vi "Pixel Manipulation.vi"() -> (3 "ImgOut":T1(plugin-control))   [LabVIEW 2014]
doc: "Use this template to build a VI to use as a subVI."
uses:
  <vilib>/vision/NI_Vision_Development_Module.lvlib
panel:
  out "FilledImg":T1(plugin-control)
  out "Pixels (U8)\nCol=50":u8[](array[numeric])
  out "Pixel Value (U8)\n(200,200)":u8
  # ":: MVi Framework V1.0 ::\nAuthor:Gaoke Yang\nEmail: gaoke.yang@yahoo.com\nWeb: www.mvicontrol.com\nCopyright (C) 2015, MVI Technologies All Rights Reserved"
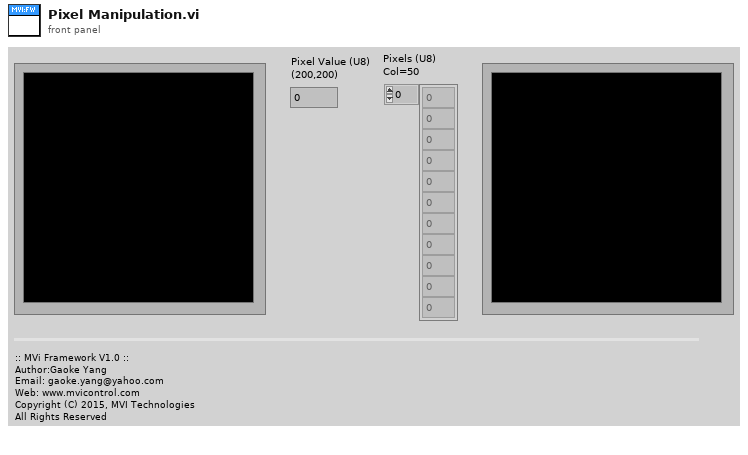
[diagram p1: front panel]
types:
  T1 = typedef "IMAQ Image.ctl" = refnum<image>
  T2 = typedef "Image Type" = u32
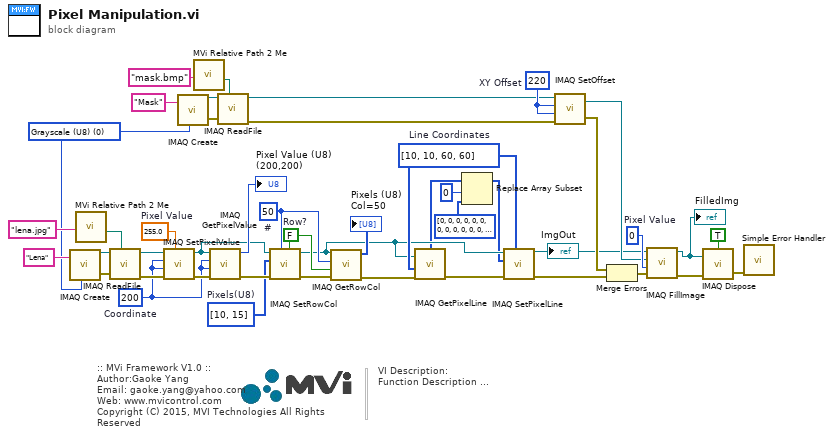
[diagram p0: block diagram]
diagram:
  w1 = u8[] [10, 15]  # Pixels(U8)
  w8 = 220  # XY Offset
  w9 = T2 0 items=["Grayscale (U8)", "Grayscale (I16)", "Grayscale (SGL)", "Complex (CSG)", "RGB (U32)", "HSL (U32)", "RGB (U64)", "Grayscale (U16)"] ("Image Type")
  w10 = 0  # Pixel Value
  w24 = i32[] [10, 10, 60, 60]  # Line Coordinates
  w28 = FALSE  # Row?
  w29 = 50  # #
  w33 = sgl 255.0  # Pixel Value
  w32 = 200  # Coordinate
  # "VI Description:\nFunction Description ..."
  # ":: MVi Framework V1.0 ::\nAuthor:Gaoke Yang\nEmail: gaoke.yang@yahoo.com\nWeb: www.mvicontrol.com\nCopyright (C) 2015, MVI Technologies All Rights Reserved"
  n1 = call "IMAQ Create"("Image Name"="Lena" ("name or relative path"), "Image Type"=w9) -> ("New Image"=w45:T1, "error out"=w44:errorcluster)  [unwired: 2 in, 1 out]
  n2 = call "MVi Relative Path 2 Me.vi"("Relative Path"="lena.jpg" ("name or relative path")) -> ("Appended Dir"=w19:path)  [unwired: 5 in, 1 out]
  n3 = call "IMAQ ReadFile"("File Path"=w19, "error in (no error)"=w44, "Image"=w45) -> ("error out"=w39:errorcluster, "Image Out"=w34:T1)  [unwired: 4 in, 3 out]
  n4 = call "IMAQ SetPixelValue"("Pixel Value"=w33, "error in (no error)"=w39, "Y Coordinate"=w32, "X Coordinate"=w32, "Image"=w34) -> ("error out"=w37:errorcluster, "Image Out"=w30:T1)  [unwired: 5 in]
  n5 = call "IMAQ Create"("Image Name"="Mask" ("name or relative path"), "Image Type"=w9) -> ("New Image"=w14:T1, "error out"=w15:errorcluster)  [unwired: 2 in, 1 out]
  n6 = call "MVi Relative Path 2 Me.vi"("Relative Path"="mask.bmp" ("name or relative path")) -> ("Appended Dir"=w12:path)  [unwired: 5 in, 1 out]
  n7 = call "IMAQ GetPixelValue"("Image"=w30, "X Coordinate"=w32, "Y Coordinate"=w32, "error in (no error)"=w37) -> ("Pixel Value (U8)"=→"Pixel Value (U8)\n(200,200)":u8, "error out"=w36:errorcluster)  [unwired: 2 in, 3 out]
  n8 = call "IMAQ ReadFile"("File Path"=w12, "error in (no error)"=w15, "Image"=w14) -> ("error out"=w6:errorcluster, "Image Out"=w7:T1)  [unwired: 4 in, 3 out]
  n9 = call "IMAQ SetRowCol"("Row / Column (Row)"=w28, "Number"=w29, "error in (no error)"=w36, "Pixels (U8)"=w1, "Image"=w30) -> ("error out"=w35:errorcluster, "Image Out"=w23:T1)  [unwired: 5 in]
  n10 = call "IMAQ GetRowCol"("Image"=w23, "Number"=w29, "Row / Column (Row)"=w28, "error in (no error)"=w35) -> ("Pixels (U8)"=→"Pixels (U8)\nCol=50":u8[], "error out"=w26:errorcluster)  [unwired: 2 in, 3 out]
  n11 = call "IMAQ GetPixelLine"("error in (no error)"=w26, "Line Coordinates"=w24, "Image"=w23) -> ("error out"=w25:errorcluster, "Pixels Line (U8)"=w22:u8[])  [unwired: 1 in, 3 out]
  n12 = Replace Array Subset(array=w22, new element=i32[] [0, 0, 0, 0, 0, 0, 0, 0, 0, 0, 0, 0, 0, 0, 0, 0, 0, 0, 0, 0, 0, 0, 0, 0, 0, 0, 0, 0, 0, 0, 0, 0, 0, 0, 0, 0, 0, 0, 0, 0, 0, 0, 0, 0, 0, 0, 0, 0, 0, 0, 0, 0, 0, 0, 0, 0, 0, 0, 0, 0, 0, 0, 0, 0, 0, 0, 0, 0, 0, 0, 0, 0, 0, 0, 0, 0, 0, 0, 0, 0, 0, 0, 0, 0, 0, 0, 0, 0, 0, 0, 0, 0, 0, 0, 0, 0, 0, 0, 0, 0, 0], index=u8 0 ("new element/subarray")) -> (w21:u8[])
  n13 = call "IMAQ SetPixelLine"("Line Coordinates"=w24, "error in (no error)"=w25, "Pixels Line (U8)"=w21, "Image"=w23) -> ("error out"=w4:errorcluster, "Image Out"=w2:T1)  [unwired: 6 in]
  "ImgOut" <- w2
  n14 = call "IMAQ SetOffset"("error in (no error)"=w6, "Y Offset"=w8, "X Offset"=w8, "Image"=w7) -> ("error out"=w5:errorcluster, "Image Out"=w3:T1)
  n15 = Merge Errors(w5, w4) -> (w11:errorcluster)
  n16 = call "IMAQ FillImage"("error in (no error)"=w11, "Pixel Value (U8, U16, I16, Float)"=w10, "Image Mask"=w3, "Image"=w2) -> ("error out"=w38:errorcluster, "Image Out"=w17:T1)  [unwired: 6 in]
  "FilledImg" <- w17
  n17 = call "IMAQ Dispose"("All Images? (No)"=TRUE, "Image"=w17, "error in (no error)"=w38) -> ("error out"=w40:errorcluster)  [unwired: 3 out]
  n18 = call <vilib>:"Simple Error Handler.vi"("error in (no error)"=w40) -> ()  [unwired: 1 in, 8 out]
